vi "RTM - Remove Unbound Channels Dependency.vi"(8 "error in (no error)":errorcluster, 9 "Menu hierarchy in":string[](array[string]), 11 "Node Ptr":u64 format="%.0x") -> (0 "error out":errorcluster, 1 "Menu hierarchy out":string[](array[string]), 3 "Action":T1)   [LabVIEW 2019, in "UDP-Custom-Device System Explorer.lvlib"]
uses:
  UDP-Custom-Device System Explorer.lvlib
  <vilib>/NI VeriStand/Custom Device API/Custom Device RTM Dependency.ctl
  Property Accessors/Shared Packet Accessors.lvlib
  <vilib>/NI VeriStand/Custom Device API/Custom Device API.lvlib
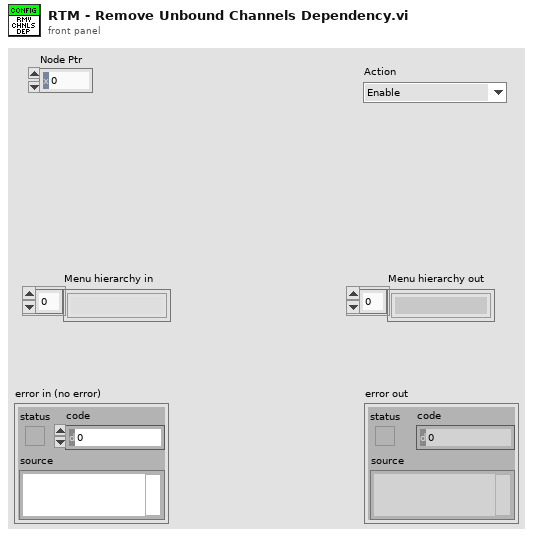
[diagram p1: front panel]
types:
  T1 = typedef "Custom Device API.lvlib/Custom Device RTM Dependency.ctl" = enum16{"Enable", "Disable", "Hide"}
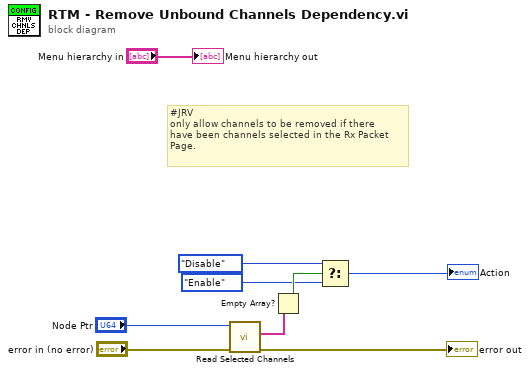
[diagram p0: block diagram]
diagram:
  # "#JRV\nonly allow channels to be removed if there\nhave been channels selected in the Rx Packet\nPage."
  n1 = call "Read Selected Channels.vi"("error in (no error)"="error in (no error)", "Node Ptr"="Node Ptr") -> ("error out"=→"error out":errorcluster, "Selected Channel Names"=w6:string[])  [unwired: 7 in, 1 out]
  n2 = Empty Array?(array=w6) -> (empty?=w5:bool)
  n3 = Select(t=Custom_Device_RTM_Dependency."Disable" ("Action"), s=w5, f=Custom_Device_RTM_Dependency."Enable" ("Action")) -> (s? t:f=→"Action":T1)
  "Menu hierarchy out" <- "Menu hierarchy in"
